vi "check_depth_sweep_parameters.vi"(8 "error in (no error)":errorcluster, 10 "Modulatin Depth Sweep Parameters":T1={"f (Hz)"=200.0, "Number of steps"=2, "Total time (s)"=2.0, "Amplitude (V)"=1.0, "depth_start (0.0 %)"=50.0, "Channel (1:Channel 1)"=2, "fc (Hz)"=2000.0, "DC Offset (V)"=0.0, "depth_end (0.0 %)"=50.0} {"depth_end (0.0 %)" min=0.0 max=120.0 format="%.1f"; "DC Offset (V)" min=-20.0 max=20.0 format="%#_13g"; "fc (Hz)" min=0.0; "Channel (1:Channel 1)" items=["Channel 1"=1, "Channel 2"=2]; "depth_start (0.0 %)" min=0.0 max=120.0 format="%.1f"; "Amplitude (V)" min=0.0 max=20.0 format="%#_13g"; "Total time (s)" min=0.0; "Number of steps" min=2; "f (Hz)" min=0.0}) -> (0 "error out":errorcluster, 1 "Array":dbl[](array[numeric]), 2 "Entered Values OK":bool)   [LabVIEW 2024, in "Sweep.lvlib"]
uses:
  Sweep.lvlib
  Type Definitions/Depth_sweep Parameters.ctl
panel:
  out "fc (Hz)":dbl
  out "Number of frequencies":i32
  out "Total time T (s)":dbl
  out "Channel (1:Channel 1)":i32
  out "Modulation Depth (0.0 %)":dbl
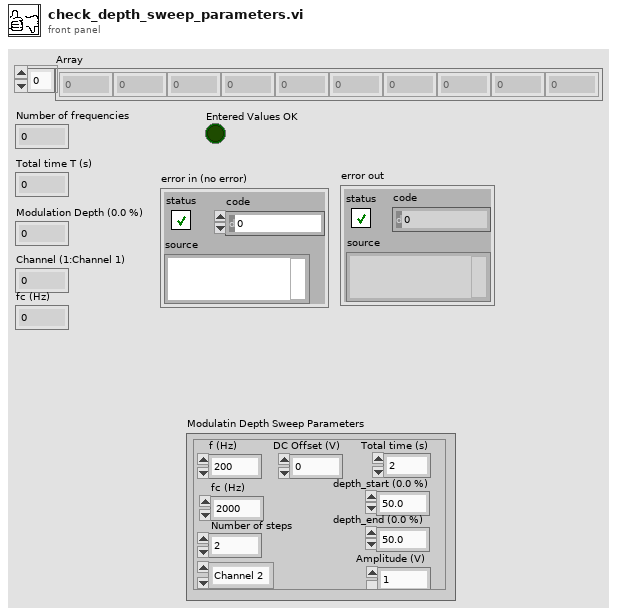
[diagram p1: front panel]
types:
  T1 = typedef "Depth_sweep Parameters.ctl" = cluster{"f (Hz)":dbl, "Number of steps":i32, "Total time (s)":dbl, "Amplitude (V)":dbl, "depth_start (0.0 %)":dbl, "Channel (1:Channel 1)":i32, "fc (Hz)":dbl, "DC Offset (V)":dbl, "depth_end (0.0 %)":dbl}
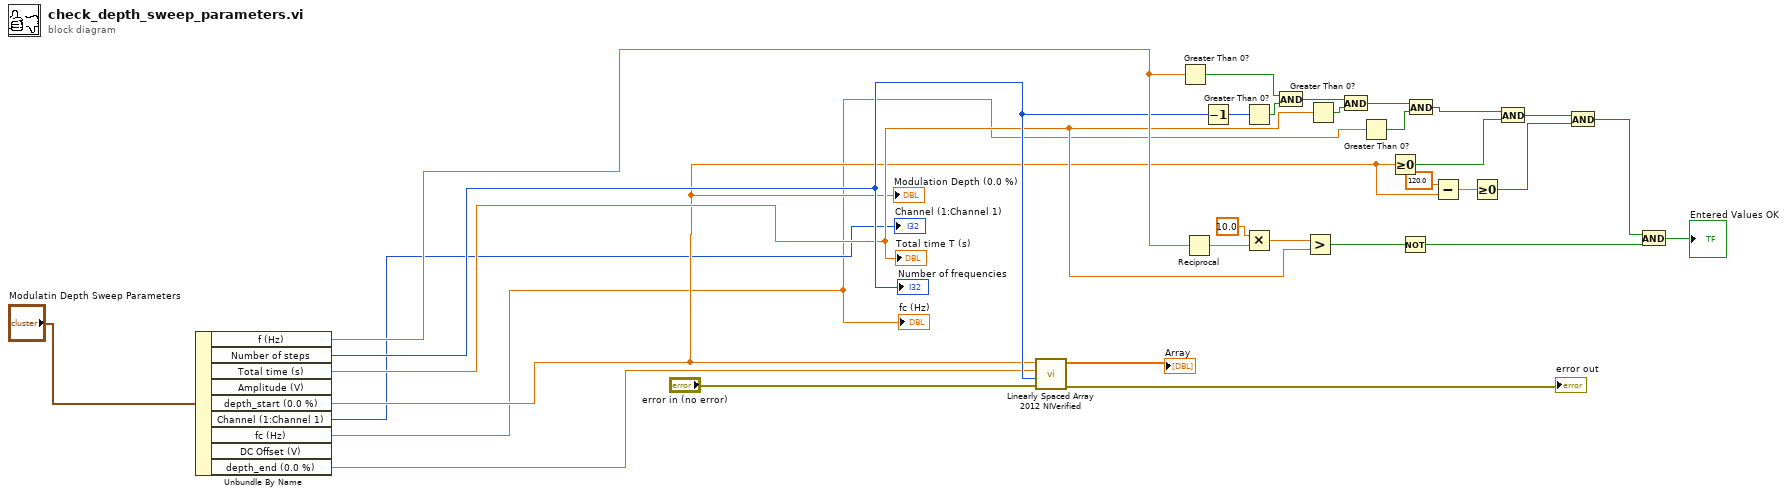
[diagram p0: block diagram]
diagram:
  n1 = Unbundle By Name("Modulatin Depth Sweep Parameters") -> ("f (Hz)"=w7:dbl, "Number of steps"=w6:i32, "Total time (s)"=w5:dbl, "depth_start (0.0 %)"=w3:dbl, "Channel (1:Channel 1)"=→"Channel (1:Channel 1)":i32, "fc (Hz)"=w1:dbl, "depth_end (0.0 %)"=w4:dbl)  [unwired: 2 out]
  "Modulation Depth (0.0 %)" <- w3
  "Total time T (s)" <- w5
  "Number of frequencies" <- w6
  "fc (Hz)" <- w1
  n2 = call "Linearly Spaced Array 2012 NIVerified.vi"("error in (no error)"="error in (no error)", "Number of Samples"=w6, "End"=w4, "Start"=w3) -> ("error out"=→"error out":errorcluster, "Array"=→"Array":dbl[])  [unwired: 6 in]
  n3 = Greater Than 0?(x=w7) -> (x > 0?=w22:bool)
  n4 = Reciprocal(x=w7) -> (1/x=w10:dbl)
  n5 = Decrement(x=w6) -> (x-1=w18:i32)
  n6 = Greater Than 0?(x=w18) -> (x > 0?=w23:bool)
  n7 = Multiply(x=10.0, y=w10) -> (x*y=w29:dbl)
  n8 = And(x=w22, y=w23) -> (x .and. y?=w24:bool)
  n9 = Greater?(x=w29, y=w5) -> (0:w30:bool)
  n10 = Greater Than 0?(x=w5) -> (x > 0?=w25:bool)
  n11 = And(x=w24, y=w25) -> (x .and. y?=w26:bool)
  n12 = Greater Than 0?(x=w1) -> (x > 0?=w27:bool)
  n13 = Greater Or Equal To 0?(x=w3) -> (x >= 0?=w17:bool)
  n14 = Not(x=w30) -> (.not. x?=w31:bool)
  n15 = And(x=w26, y=w27) -> (x .and. y?=w11:bool)
  n16 = Subtract(x=120.0, y=w3) -> (x-y=w14:dbl)
  n17 = Greater Or Equal To 0?(x=w14) -> (x >= 0?=w13:bool)
  n18 = And(x=w11, y=w17) -> (x .and. y?=w15:bool)
  n19 = And(x=w15, y=w13) -> (x .and. y?=w16:bool)
  n20 = And(x=w16, y=w31) -> (x .and. y?=→"Entered Values OK":bool)
